vi "Translation3d_Plus.vi"(9 "other Translation3d":T1 {"Z" format="%14.3f"; "Y" format="%14.3f"; "X" format="%14.3f"}, 11 "In Translation3d":T1 {"Z" format="%14.3f"; "Y" format="%14.3f"; "X" format="%14.3f"}) -> (3 "Out Translation3d":T1 {"Z" format="%14.3f"; "Y" format="%14.3f"; "X" format="%14.3f"})   [LabVIEW 2019, in "Trajectory_Library.lvlib"]
doc: "Adds two translations in 2d space and returns the sum. This is similar to vector addition.\n \nFor example, Translation2d{1.0, 2.5} + Translation2d{2.0, 5.5} = Translation2d{3.0, 8.0}\n\nParameters:\n - IN Translation - This translation data structure\n - other Translation - The translation data structure to add\n\nReturns\n - Out Translation - The summation of the two translations."
uses:
  Trajectory_Library.lvlib
  TRANSLATION3D.ctl
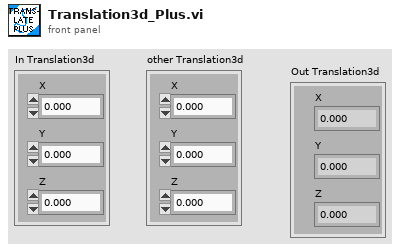
[diagram p1: front panel]
types:
  T1 = typedef "Trajectory_Library.lvlib/TRANSLATION3D.ctl" = cluster{"X":dbl, "Y":dbl, "Z":dbl}
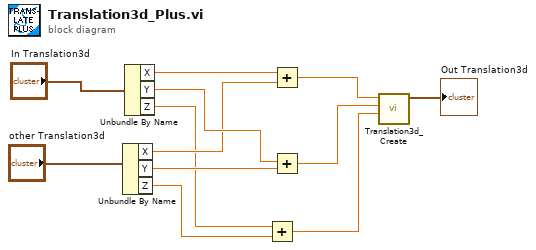
[diagram p0: block diagram]
diagram:
  n1 = Unbundle By Name("other Translation3d") -> ("X"=w3:dbl, "Y"=w9:dbl, "Z"=w1:dbl)
  n2 = Unbundle By Name("In Translation3d") -> ("X"=w10:dbl, "Y"=w8:dbl, "Z"=w2:dbl)
  n3 = Add(x=w2, y=w1) -> (x+y=w4:dbl)
  n4 = Add(x=w10, y=w3) -> (x+y=w7:dbl)
  n5 = Add(x=w8, y=w9) -> (x+y=w6:dbl)
  n6 = call "Translation3d_Create.vi"("Z"=w4, "Y"=w6, "X"=w7) -> ("TRANSLATION3D"=→"Out Translation3d":T1)  [unwired: 8 in]
